vi "Add No Connections Error.vi"(6 "pin type":T1, 8 "error in":errorcluster, 9 "instrument type id":string, 10 "site":i32, 11 "pin or relay names":string[](array[string])) -> (0 "error out":errorcluster)   [LabVIEW 2020, in "Measurement Plugin Session Management V1.lvlib" / "Session Reservation.lvclass"]
uses:
  Session Reservation.lvclass
  Pin Type.ctl
  Measurement Plugin Measurement Server/Helpers/Error Strings Global Internal.vi
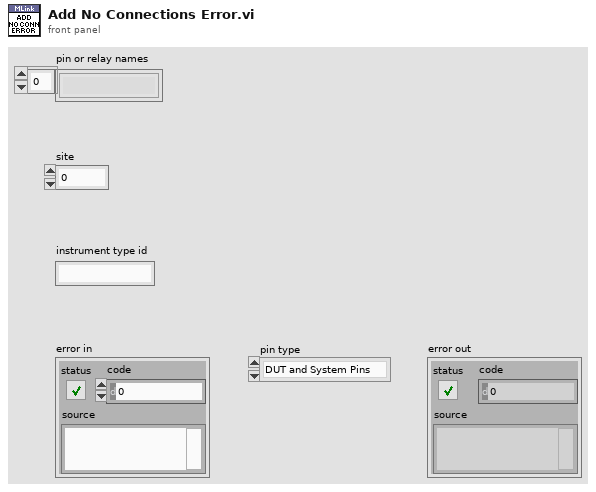
[diagram p1: front panel]
types:
  T1 = typedef "Measurement Plugin Session Management V1.lvlib/Session Reservation.lvclass/Pin Type.ctl" = enum16{"DUT and System Pins", "System Pins"}
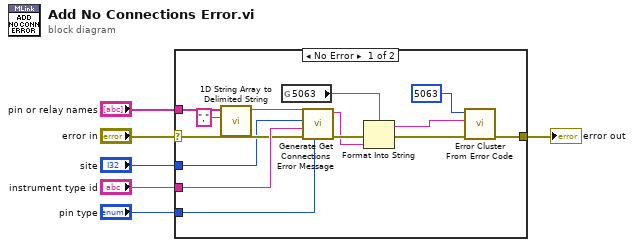
[diagram p0: block diagram]
diagram:
  n1 = case shown="No Error" "error in" {
    selector: "error in" -> [w11 w21]
    tunnel: [w20 w21] -> w5
    tunnel: "pin or relay names" -> [w15 _]
    tunnel: "site" -> [w9 _]
    tunnel: "instrument type id" -> [w13 _]
    tunnel: "pin type" -> [w7 _]
    frame No Error {
      n2 = call <vilib>:"1D String Array to Delimited String.vi"("delimiter"=",", "string array"=w15) -> ("delimited string"=w10:string)  [unwired: 9 in]
      n3 = global read "Error Strings Global Internal.vi" "5063"() -> (w19:string)
      n4 = call "Generate Get Connections Error Message.vi"("pin type"=w7, "error in"=w11, "instrument type id"=w13, "site"=w9, "pin or relay names"=w10) -> ("error out"=w12:errorcluster, "error string"=w8:string)  [unwired: 5 in]
      n5 = Format Into String(format string=w19, error in=w12, w8) -> (resulting string=w16:string, error out=w18:errorcluster)  [unwired: 1 in]
      n6 = call <vilib>:"Error Cluster From Error Code.vi"("error in (no error)"=w18, "error message (\"\")"=w16, "error code (0)"=5063) -> ("error out"=w20:errorcluster)  [unwired: 6 in]
    }
    frame Error {
    }
  }
  "error out" <- w5
